vi "Create.vi"(8 "error in (no error)":errorcluster) -> (0 "error out":errorcluster, 3 "Mock Class Generator out":refnum<class "Test Interface Mock.lvclass">)   [LabVIEW 2020, in "Test Interface Mock.lvclass"]
uses:
  Test Interface Mock.lvclass
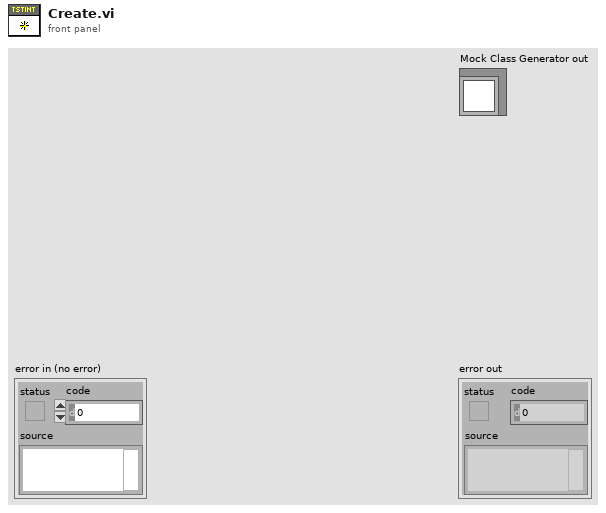
[diagram p1: front panel]
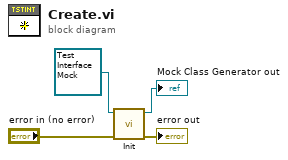
[diagram p0: block diagram]
diagram:
  n1 = call-dynamic "Init.vi"("error in (no error)"="error in (no error)", "Mock In"=refnum<class "Test Interface Mock.lvclass"> refnum ("Mock in")) -> ("error out"=→"error out":errorcluster, "Mock Out"=→"Mock Class Generator out":refnum<class "Test Interface Mock.lvclass">)  [unwired: 8 in]
